vi "Calculate time to acquire stack.vi"(8 "error in (no error)":errorcluster, 11 "Tomo in":refnum<class "Invivo_Tomo.lvclass">) -> (0 "error out":errorcluster, 3 "Tomo out":refnum<class "Invivo_Tomo.lvclass">)   [LabVIEW 2012, in "Invivo_Tomo.lvclass"]
uses:
  Invivo_Tomo.lvclass
  Invivo_Tomo.lvclass/Invivo_Tomo.ctl
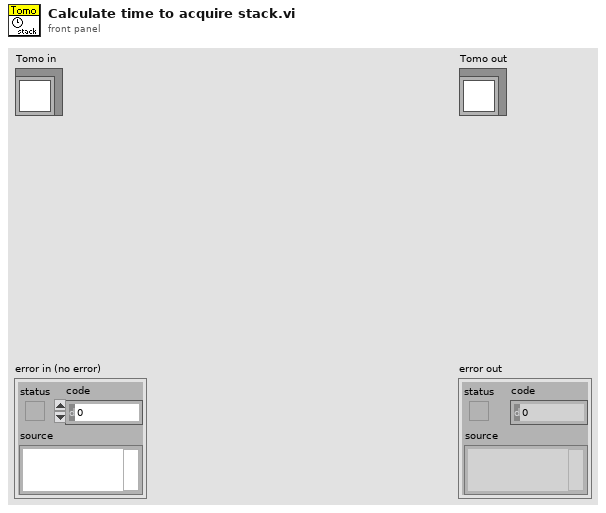
[diagram p1: front panel]
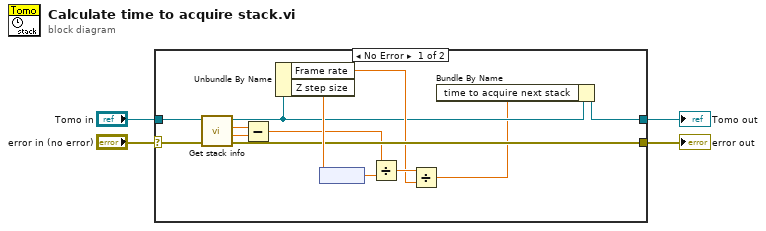
[diagram p0: block diagram]
diagram:
  n1 = case shown="No Error" "error in (no error)" {
    selector: "error in (no error)" -> [w12 w19]
    tunnel: [w11 w19] -> w3
    tunnel: [w6 w18] -> w1
    tunnel: "Tomo in" -> [w13 w18]
    frame No Error {
      n2 = call-dynamic "Get stack info.vi"("error in (no error)"=w12, "Tomo in"=w13) -> ("error out"=w11:errorcluster, "Z start"=w16:dbl, "Z stop"=w17:dbl, "Tomo out"=w7:refnum<class "Invivo_Tomo.lvclass">)  [unwired: 4 in, 2 out]
      n3 = Subtract(x=w17, y=w16) -> (x-y=w10:dbl)
      n4 = Unbundle By Name(w7) -> ("Frame rate"=w8:dbl[unit], "Z step size"=w15:dbl[unit])
      n5 = node(w15) -> (w14:dbl)
      n6 = Divide(x=w10, y=w14) -> (x/y=w9:dbl)
      n7 = Divide(x=w9, y=w8) -> (x/y=w5:dbl[unit])
      n8 = Bundle By Name(cluster=w7, "time to acquire next stack"=w5) -> (w6:refnum<class "Invivo_Tomo.lvclass">)
    }
    frame Error {
    }
  }
  "error out" <- w3
  "Tomo out" <- w1
